vi "Enqueue.vi"(8 "error in":errorcluster, 10 "Data":variant, 11 "State":T1) -> (0 "error out":errorcluster)   [LabVIEW 2018, in "Entry Console.lvlib"]
uses:
  Entry Console.lvlib
  ctl/Module State.ctl
  ctl/Queue Actions.ctl
  ctl/Module Message.ctl
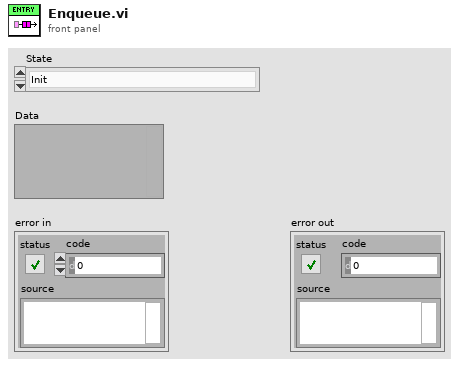
[diagram p1: front panel]
types:
  T1 = typedef "Entry Console.lvlib/Module State.ctl" = enum16{"Init", "Idle", "Error", "Close", "Wash Step Selection Buttons: Enable/Disable All", "Wash Step Selection Buttons: Set All", "Wash Step Selection Buttons: Set Single (On/Off)", "Start: Enable/Disable", "Start: Set State (On/Off)"}
  T2 = typedef "Entry Console.lvlib/Module Message.ctl" = cluster{"State":T1, "Data":variant}
  T3 = typedef "Entry Console.lvlib/Queue Actions.ctl" = enum16{"Create", "Get", "Destroy"}
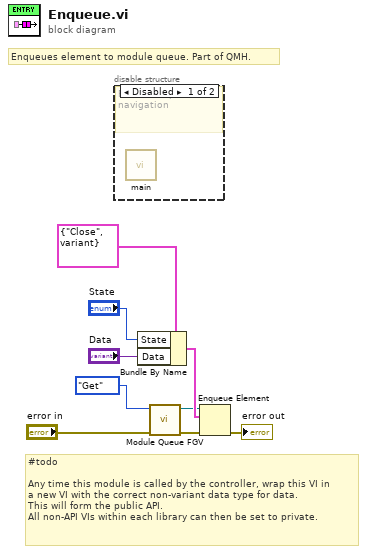
[diagram p0: block diagram]
diagram:
  # "#todo\n\nAny time this module is called by the controller, wrap this VI in\na new VI with the correct non-variant data type for data. \nThis will form the public API.\nAll non-API VIs within each library can then be set to private."
  # "Enqueues element to module queue. Part of QMH."
  n1 = disable-structure shown="Disabled" {
    frame Disabled {
      # "For Developer - \nnavigation"
      n2 = call "main.vi"() -> ()  [unwired: 11 in, 1 out]
    }
    frame Enabled {
    }
  }
  n3 = Bundle By Name(cluster=T2 {"State"=enum."Close", "Data"=variant} ("element"), "State"="State", "Data"="Data") -> (w6:T2)
  n4 = call "Module Queue FGV.vi"("error in"="error in", "Action"=Queue_Actions."Get") -> ("error out"=w4:errorcluster, "Queue ref"=w3:refnum<queue>)  [unwired: 8 in]
  n5 = Enqueue Element(queue=w3, element=w6, error in (no error)=w4) -> (error out=→"error out":errorcluster)  [unwired: 1 in, 2 out]
